vi "Sig2MS SignalToPy.vi"(7 "getType":enum16{"All", "Spectra", "Ionisation"}(ring), 8 "error in (no error)":errorcluster, 10 "rawSignal":waveform(sgl)) -> (0 "error out":errorcluster, 3 "pySigFormat":T1)   [LabVIEW 2018, in "Sig2MS.lvclass"]
uses:
  Sig2MS.lvclass
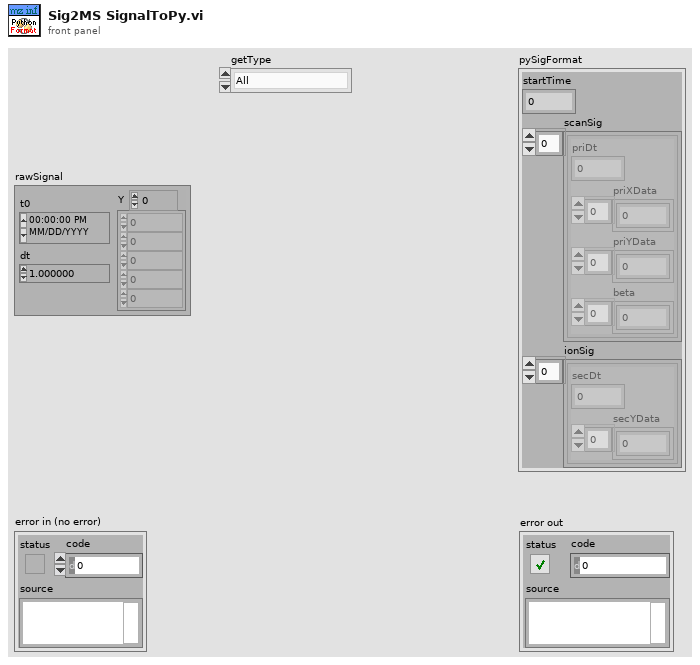
[diagram p1: front panel]
types:
  T1 = cluster{"startTime":dbl, "scanSig":cluster{"priDt":dbl, "priXData":dbl[], "priYData":sgl[], "beta":dbl[]}[], "ionSig":cluster{"secDt":dbl, "secYData":sgl[]}[]}
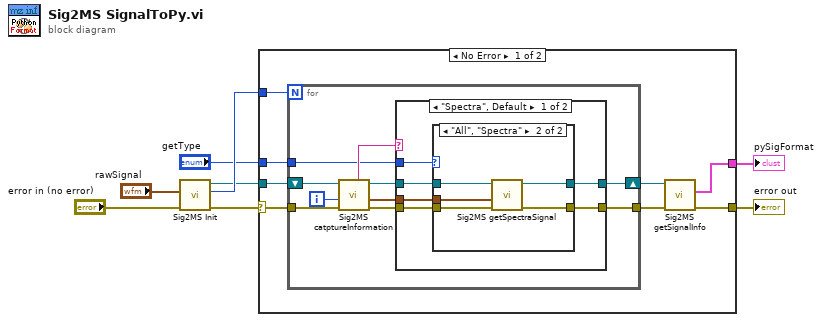
[diagram p0: block diagram]
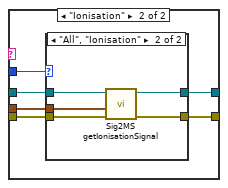
[diagram p3: hidden frame]
diagram:
  n1 = call "Sig2MS Init.vi"("error in (no error)"="error in (no error)", "signal in"="rawSignal") -> ("error out"=w6:errorcluster, "Size"=w5:i32, "Sig2MS out"=w4:refnum<class "Sig2MS.lvclass">)  [unwired: 7 in]
  n2 = case shown="No Error" w6 {
    selector: w6 -> [w11 w53]
    tunnel: w5 -> [w15 _]
    tunnel: w4 -> [w16 _]
    tunnel: "getType" -> [w14 _]
    tunnel: [w10 w53] -> w2
    tunnel: [w9 _] -> w1
    frame No Error {
      n3 = for {
        N: w15 -> [_]
        shift-right: [w25] -> w13
        shift-left: w16 -> [w26]
        tunnel: [w24] -> w12
        tunnel: w14 -> [w18]
        tunnel: w11 -> [w17]
        i -> [w23]
        n4 = call "Sig2MS catptureInformation.vi"("error in (no error)"=w17, "Index"=w23, "Sig2MS in"=w26) -> ("error out"=w19:errorcluster, "SectionalSig"=w20:waveform(sgl), "Sig2MS out"=w21:refnum<class "Sig2MS.lvclass">, "Label"=w22:string)  [unwired: 5 in]
        n5 = case shown="\"Spectra\", Default" w22 {
          tunnel: w19 -> [w28 w41]
          tunnel: w21 -> [w30 w43]
          tunnel: w20 -> [w29 w42]
          tunnel: [w32 w45] -> w25
          tunnel: [w31 w44] -> w24
          tunnel: w18 -> [w27 w40]
          frame "Spectra", Default {
            n6 = case shown="\"All\", \"Spectra\"" w27 {
              tunnel: [w34 w39] -> w32
              tunnel: [w33 w38] -> w31
              tunnel: w30 -> [w34 w37]
              tunnel: w29 -> [_ w36]
              tunnel: w28 -> [w33 w35]
              frame "Ionisation", Default {
              }
              frame "All", "Spectra" {
                n7 = call "Sig2MS getSpectraSignal.vi"("error in (no error)"=w35, "signal in"=w36, "Sig2MS in"=w37) -> ("error out"=w38:errorcluster, "Sig2MS out"=w39:refnum<class "Sig2MS.lvclass">)  [unwired: 7 in]
              }
            }
          }
          frame "Ionisation" {
            n8 = case shown="\"All\", \"Ionisation\"" w40 {
              tunnel: [w47 w48] -> w45
              tunnel: [w46 w49] -> w44
              tunnel: w43 -> [w47 w52]
              tunnel: w42 -> [_ w51]
              tunnel: w41 -> [w46 w50]
              frame "Spectra", Default {
              }
              frame "All", "Ionisation" {
                n9 = call "Sig2MS getIonisationSignal.vi"("error in (no error)"=w50, "signal in"=w51, "Sig2MS in"=w52) -> ("error out"=w49:errorcluster, "Sig2MS out"=w48:refnum<class "Sig2MS.lvclass">)  [unwired: 7 in]
              }
            }
          }
        }
      }
      n10 = call "Sig2MS getSignalInfo.vi"("error in (no error)"=w12, "Sig2MS in"=w13) -> ("error out"=w10:errorcluster, "pySigFormat"=w9:T1)  [unwired: 7 in, 1 out]
    }
    frame Error {
    }
  }
  "error out" <- w2
  "pySigFormat" <- w1
